vi "Sys config window-Get set control values.vi"(8 "error in (no error)":errorcluster, 11 "Function":T33) -> (0 "error out":errorcluster, 3 "output cluster":T1={"Triggers output setup"=[], "General trigger settings"={"Trigger 1 function"=enum."Encoder trigger", "Triggers loop clock (MHz)"=80.0}, "Calibration settings"={"Pockels cal.Zoom"=0, "Pockels cal.Dwell time (µs)"=0.0}, "Hardware Configuration"={"Dev. PC"=FALSE, "Swap XY on stage"=FALSE, "No of AOD"=0, "MC Supported"=FALSE, "Axial MC"=FALSE, "Computer MAC address"="", "Externalise Triggers"=FALSE, "Trigger HW config"={"Available Device List"=0, "Device Address"=""}, "DAQmx Chan"={"Pockels AO"="", "Hard shutter AO"="", "PMT AOs"="", "Galvo AOs"="", "Power meter AI"=""}, "XYZ Stage Control Config"=enum."None", "XY stage available"=FALSE, "XY Comms Config Cluster"={"Name"="", "Device Address"="", "Port "=0, "Baudrate"=0, "Comms Type"=enum."GPIB-IEEE488"}, "Y stage available"=FALSE, "Y Comms Config Cluster"={"Name"="", "Device Address"="", "Port "=0, "Baudrate"=0, "Comms Type"=enum."GPIB-IEEE488"}, "Z stage available"=FALSE, "Z Comms Config Cluster "={"Name"="COM7", "Device Address"="", "Port "=0, "Baudrate"=0, "Comms Type"=enum."GPIB-IEEE488"}, "Encoder available"=FALSE, "Encoder"={"IP address"="224.0.1.103", "Port"=7000, "Wheel radius (cm)"=16.0, "Encoder Trigger"=""}, "VidRec available"=FALSE, "Cam VidRec"={"DO flag-Video record"="", "DO flag-Trial start"=""}, "Laser Power Control HW config"={"Laser Power Control"="", "Laser Power Modulation Control"=enum."NI"}, "Laser 1 available"=FALSE, "Laser 1 config cluster"={"COM port"="COM7", "Baud Rate"=0, "Type"=""}, "Prechirper 1 available"=FALSE, "Prechirper 1 config cluster"={"Type"="", "Baud Rate"=0, "COM port"="COM7"}, "Control system.FPGA available?"=FALSE, "Control Sys. HW config"={"Control system.FPGA Type"=enum."Virtex 5", "Control system.Network adapter name"="", "Control system.MAC address"="", "Control system.Ethernet Port"=0, "Control system.Ethernet Port Opened"=FALSE}, "DAQ FPGA HW Config"={"FGPA Ref"=refnum, "Target"="RIO0", "input card type"=enum."AC Card"}, "PMT Control Voltage Limits"={"Lower Limit"=0.0, "Upper Limit"=0.0}}, "System Config"={"Laser wavelength (nm)"=920.0, "DAQ FPGA System"={"Clock Freq (MHz) "=200.0, "Samples Wait after Trigger"=5080, "AOD fill"=4900, "StartupDelay"=0, "Slip Cycle (clock cycles)"=600000, "Add Cycle"=TRUE}, "Control system"={"AOD 1 Amplitude"=0, "AOD 2 Amplitude"=0, "AOD 3 Amplitude"=0, "AOD 4 Amplitude"=0, "AOD 5 Amplitude"=0, "AOD 6 Amplitude"=0, "T0 (ns)"=0.0, "Ta (ns)"=0.0, "Data Time Interval (ns)"=0.0, "Ctrl FPGA Clock (MHz)"=240.0}}, "Calibration config."={"Current Objective"="", "Objective Settings"=[], "PreChirper Values Preset ?"=FALSE, "PreChirper Settings"=[], "PreChirper Constants"={"a 1"=0, "b 1"=0, "c 1"=0, "a 2"=0, "b 2"=0, "c 2"=0, "lmin"=0, "lmax"=0}}, "General Setup"={"Microscope ID"="003", "Microscope Type"="AOLM", "Revision Number"="1.0.0.0", "Advanced Imaging"=FALSE, "Error Logging"=FALSE, "Performance Monitoring"=FALSE, "Max Allowed Trial Length"=60.0, "Initial Scan Resolution"=512.0, "Initial Acceptance Angle"=5.0, "Initial Laser Wavelength"=900.0, "Initial Dwell Time"=900.0}, "AOD Settings - distilled"={"AOD 1 thickness (mm)"=8.0, "AOD 2 thickness (mm)"=8.0, "AOD 3 thickness (mm)"=8.0, "AOD 4 thickness (mm)"=8.0, "AOD 1-2 separation (mm)"=50.0, "AOD 2-3 separation (mm)"=50.0, "AOD 3-4 separation (mm)"=50.0, "AOD 1 Centre (mm)"=7.5, "AOD 2 Centre (mm)"=7.5, "AOD 3 Centre (mm)"=7.5, "AOD 4 Centre (mm)"=7.5, "AOD 1 X Offset"=0.0, "AOD 2 X Offset"=0.0023, "AOD 3 X Offset"=0.0046, "AOD 4 X Offset"=0.0046, "AOD 1 Y Offset"=0.0, "AOD 2 Y Offset"=0.0, "AOD 3 Y Offset"=0.0023, "AOD 4 Y Offset"=0.0046, "Timing Offset AOD 1"=0.0, "Timing Offset AOD 2"=0.0, "Timing Offset AOD 3"=0.0, "Timing Offset AOD 4"=0.0, "AOL centre wavelength (nm)"=1.0, "AOL centre frequency (MHz)"=1.0, "Pair deflection ratio"=1.0, "AOL aperture (mm)"=15.0, "AOD fill time (us)"=1.0, "Diffraction mode"=1.0, "Crystal length (mm)"=0.0, "Acoustic velocity (m/s)"=1.0, "AOD Ord. Refractive index"=2.22}} {"System Config"."Control system"."Ctrl FPGA Clock (MHz)" min=80.0 max=500.0 step=1.0; "System Config"."Control system"."Data Time Interval (ns)" min=0.0 max=2048.0 step=1.0; "System Config"."Control system"."Ta (ns)" min=0.0 max=2048.0 step=1.0; "System Config"."Control system"."T0 (ns)" min=0.0 max=2048.0 step=1.0; "System Config"."Control system"."AOD 6 Amplitude" min=0 max=2048 step=1; "System Config"."Control system"."AOD 5 Amplitude" min=0 max=2048 step=1; "System Config"."Control system"."AOD 4 Amplitude" min=0 max=2048 step=1; "System Config"."Control system"."AOD 3 Amplitude" min=0 max=2048 step=1; "System Config"."Control system"."AOD 2 Amplitude" min=0 max=2048 step=1; "System Config"."Control system"."AOD 1 Amplitude" min=0 max=2048 step=1; "System Config"."Laser wavelength (nm)" min=800.0 max=1080.0 step=1.0; "Hardware Configuration"."Encoder"."Wheel radius (cm)" format="%#_13g"; "General trigger settings"."Triggers loop clock (MHz)" format="%#_13g"; "Triggers output setup"."Pulse width (us)" min=10 max=5000 step=1 format="%.0fµs"})   [LabVIEW 2020]
uses:
  Typedefs/HW config states enum.ctl
  Globals/Sys Config window globals.vi
  Configuration code/Calibration/Globals/gl_Calibration globals.vi
  Configuration code/Typedefs/Pockels Calibration settings cluster.ctl
  Global Variables/General Globals.vi
  Peripherals Control/Triggers/Typedefs/Trigger setup element cluster.ctl
  Peripherals Control/Triggers/Typedefs/Triggers output setup.ctl
  Typedefs/Trigger 1 selector enum.ctl
  Peripherals Control/Triggers/Typedefs/General trigger settings cluster.ctl
  Typedefs/Cam VidRec HW config setup cluster.ctl
  Typedefs/Control Sys HW config cluster.ctl
  <vilib>/userDefined/High Color/nirio_resource_hc.ctl
  Typedefs/FPGA input type AC-DC.ctl
  Typedefs/DAQmx physical channels cluster.ctl
  Typedefs/Encoder config cluster.ctl
  Typedefs/Triggers HW config.ctl
  Typedefs/Laser 1 config cluster.ctl
  Typedefs/PreChirper 1 config cluster.ctl
  Typedefs/Laser Power Control HW config.ctl
  Typedefs/Hardware Configuration settings.ctl
  RIG-SPECIFIC FILES/FPGA Refs/FPGA Ref.ctl
  Typedefs/DAQ FPGA system config.ctl
  Typedefs/CTRL system config.ctl
  Typedefs/System Configuration.ctl
  Configuration code/Typedefs/Initial config.ctl
  Typedefs/PreChirper constants.ctl
  Typedefs/Prechirper Cal Config.ctl
  Typedefs/Objective Config.ctl
  Typedefs/Calibration config.ctl
  Typedefs/fgv_actions.ctl
  Typedefs/General Setup.ctl
  Typedefs/AOD Settings-distilled.ctl
  Typedefs/DAQ FPGA HW config cluster.ctl
  Typedefs/PMT Control Voltage limits.ctl
  Peripherals Control/XYZ Stage/Control/typedefs/XYZControlConfig.ctl
  Typedefs/Comms Type.ctl
  Typedefs/Peripherals comms config cluster.ctl
  Visualisation/Functional Imaging Viewer/Typedefs/Get-Set-Clear Control.ctl
panel:
  # "Thickness (mm)"
  # "X Offset"
  # "Separation (mm)"
  # "Y Offset"
  # "Centre (mm)"
  # "Timing Offset"
  # "(make , model etc)"
  # "(COM Port / IP Address / service address etc.)"
  # "(Port for ethernet / channel for BT)"
  # "(make , model etc)"
  # "(COM Port / IP Address / service address etc.)"
  # "(Port for ethernet / channel for BT)"
  # "(make , model etc)"
  # "(COM Port / IP Address / service address etc.)"
  # "(Port for ethernet / channel for BT)"
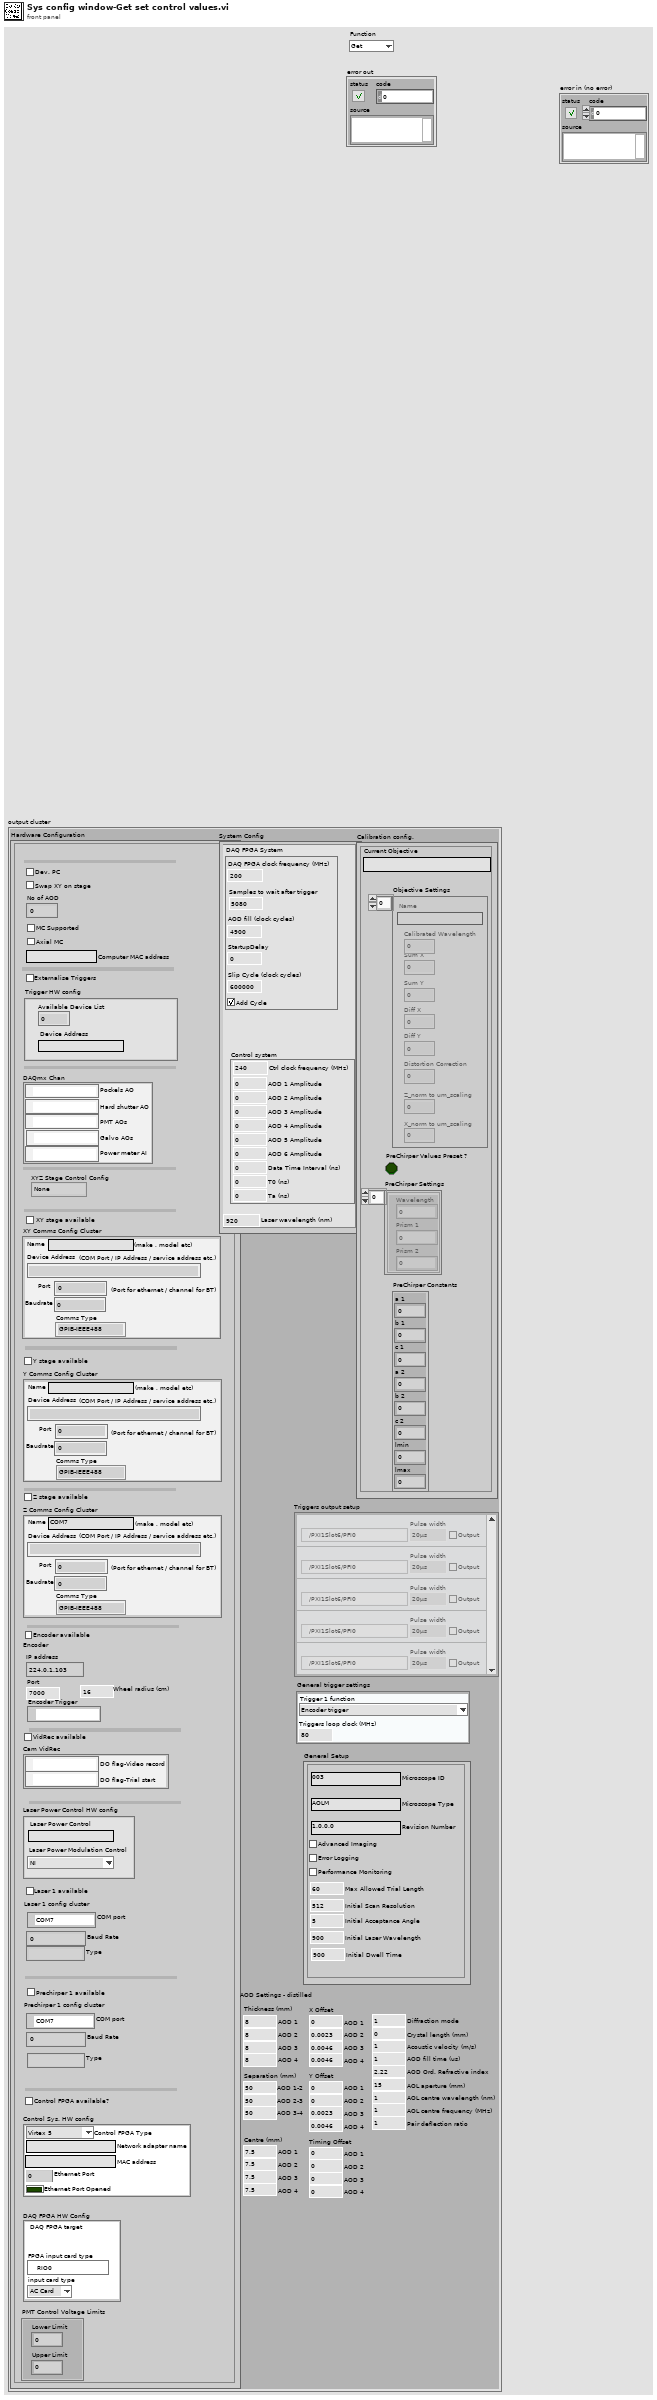
[diagram p1: front panel]
types:
  T1 = typedef "Initial config.ctl" = cluster{"Triggers output setup":T2, "General trigger settings":T4, "Calibration settings":T6, "Hardware Configuration":T7, "System Config":T24, "Calibration config.":T27, "General Setup":T31, "AOD Settings - distilled":T32}
  T2 = typedef "Triggers output setup.ctl" = T3[]
  T3 = typedef "Trigger setup element cluster.ctl" = cluster{"Name":string, "Output?":bool, "Output terminal":tag, "PXI backplane line":tag, "Pulse width (us)":u16}
  T4 = typedef "General trigger settings cluster.ctl" = cluster{"Trigger 1 function":T5, "Triggers loop clock (MHz)":dbl}
  T5 = typedef "Trigger 1 selector enum.ctl" = enum16{"Encoder trigger", "Line trigger", "Control system's ref frame acknowledgement"}
  T6 = typedef "Pockels Calibration settings cluster.ctl" = cluster{"Pockels cal.Zoom":u8, "Pockels cal.Dwell time (µs)":dbl}
  T7 = typedef "Hardware Configuration settings.ctl" = cluster{"Dev. PC":bool, "Swap XY on stage":bool, "No of AOD":u8, "MC Supported":bool, "Axial MC":bool, "Computer MAC address":string, "Externalise Triggers":bool, "Trigger HW config":T8, "DAQmx Chan":T9, "XYZ Stage Control Config":T10, "XY stage available":bool, "XY Comms Config Cluster":T11, "Y stage available":bool, "Y Comms Config Cluster":T11, "Z stage available":bool, "Z Comms Config Cluster ":T11, "Encoder available":bool, "Encoder":T13, "VidRec available":bool, "Cam VidRec":T14, "Laser Power Control HW config":T15, "Laser 1 available":bool, "Laser 1 config cluster":T16, "Prechirper 1 available":bool, "Prechirper 1 config cluster":T17, "Control system.FPGA available?":bool, "Control Sys. HW config":T18, "DAQ FPGA HW Config":T19, "PMT Control Voltage Limits":T23}
  T8 = typedef "Triggers HW config.ctl" = cluster{"Available Device List":i32, "Device Address":string}
  T9 = typedef "DAQmx physical channels cluster.ctl" = cluster{"Pockels AO":tag, "Hard shutter AO":tag, "PMT AOs":tag, "Galvo AOs":tag, "Power meter AI":tag}
  T10 = typedef "XYZControlConfig.ctl" = enum16{"None", "XYZ", "XY-Z", "X-Y-Z", "Z"}
  T11 = typedef "Peripherals comms config cluster.ctl" = cluster{"Name":string, "Device Address":string, "Port ":u16, "Baudrate":i32, "Comms Type":T12}
  T12 = typedef "Comms Type.ctl" = enum16{"GPIB-IEEE488", "Serial-RS232", "Serial-RS485", "Serial-RS422", "Serial-USB", "Ethernet-TCP/IP", "Ethernet-UDP"}
  T13 = typedef "Encoder config cluster.ctl" = cluster{"IP address":string, "Port":u16, "Wheel radius (cm)":dbl, "Encoder Trigger":tag}
  T14 = typedef "Cam VidRec HW config setup cluster.ctl" = cluster{"DO flag-Video record":tag, "DO flag-Trial start":tag}
  T15 = typedef "Laser Power Control HW config.ctl" = cluster{"Laser Power Control":string, "Laser Power Modulation Control":enum16{"NI", "FPGA"}}
  T16 = typedef "Laser 1 config cluster.ctl" = cluster{"COM port":refnum<visa-resource-name>, "Baud Rate":i32, "Type":string}
  T17 = typedef "PreChirper 1 config cluster.ctl" = cluster{"Type":string, "Baud Rate":i32, "COM port":refnum<visa-resource-name>}
  T18 = typedef "Control Sys HW config cluster.ctl" = cluster{"Control system.FPGA Type":enum16{"Virtex 5", "Virtex 7"}, "Control system.Network adapter name":string, "Control system.MAC address":string, "Control system.Ethernet Port":u32, "Control system.Ethernet Port Opened":bool}
  T19 = typedef "DAQ FPGA HW config cluster.ctl" = cluster{"FGPA Ref":T20, "Target":T21, "input card type":T22}
  T20 = typedef "FPGA Ref.ctl" = refnum<k20>
  T21 = typedef "nirio_resource_hc.ctl" = tag
  T22 = typedef "FPGA input type AC-DC.ctl" = enum16{"AC Card", "DC Card"}
  T23 = typedef "PMT Control Voltage limits.ctl" = cluster{"Lower Limit":dbl, "Upper Limit":dbl}
  T24 = typedef "System Configuration.ctl" = cluster{"Laser wavelength (nm)":dbl, "DAQ FPGA System":T25, "Control system":T26}
  T25 = typedef "DAQ FPGA system config.ctl" = cluster{"Clock Freq (MHz) ":dbl, "Samples Wait after Trigger":u16, "AOD fill":u16, "StartupDelay":i32, "Slip Cycle (clock cycles)":u32, "Add Cycle":bool}
  T26 = typedef "CTRL system config.ctl" = cluster{"AOD 1 Amplitude":i16, "AOD 2 Amplitude":i16, "AOD 3 Amplitude":i16, "AOD 4 Amplitude":i16, "AOD 5 Amplitude":i16, "AOD 6 Amplitude":i16, "T0 (ns)":dbl, "Ta (ns)":dbl, "Data Time Interval (ns)":dbl, "Ctrl FPGA Clock (MHz)":dbl}
  T27 = typedef "Calibration config.ctl" = cluster{"Current Objective":string, "Objective Settings":T28[], "PreChirper Values Preset ?":bool, "PreChirper Settings":T29[], "PreChirper Constants":T30}
  T28 = typedef "Objective Config.ctl" = cluster{"Name":string, "Sum X":dbl, "Sum Y":dbl, "Diff X":dbl, "Diff Y":dbl, "Distortion Correction":dbl, "Z_norm to um_scaling":dbl, "X_norm to um_scaling":dbl, "Calibrated Wavelength":dbl}
  T29 = typedef "Prechirper Cal Config.ctl" = cluster{"Wavelength":i32, "Prism 1":i32, "Prism 2":i32}
  T30 = typedef "PreChirper constants.ctl" = cluster{"a 1":i32, "b 1":i32, "c 1":i32, "a 2":i32, "b 2":i32, "c 2":i32, "lmin":i32, "lmax":i32}
  T31 = typedef "General Setup.ctl" = cluster{"Microscope ID":string, "Microscope Type":string, "Revision Number":string, "Advanced Imaging":bool, "Error Logging":bool, "Performance Monitoring":bool, "Max Allowed Trial Length":dbl, "Initial Scan Resolution":dbl, "Initial Acceptance Angle":dbl, "Initial Laser Wavelength":dbl, "Initial Dwell Time":dbl}
  T32 = typedef "AOD Settings-distilled.ctl" = cluster{"AOD 1 thickness (mm)":dbl, "AOD 2 thickness (mm)":dbl, "AOD 3 thickness (mm)":dbl, "AOD 4 thickness (mm)":dbl, "AOD 1-2 separation (mm)":dbl, "AOD 2-3 separation (mm)":dbl, "AOD 3-4 separation (mm)":dbl, "AOD 1 Centre (mm)":dbl, "AOD 2 Centre (mm)":dbl, "AOD 3 Centre (mm)":dbl, "AOD 4 Centre (mm)":dbl, "AOD 1 X Offset":dbl, "AOD 2 X Offset":dbl, "AOD 3 X Offset":dbl, "AOD 4 X Offset":dbl, "AOD 1 Y Offset":dbl, "AOD 2 Y Offset":dbl, "AOD 3 Y Offset":dbl, "AOD 4 Y Offset":dbl, "Timing Offset AOD 1":dbl, "Timing Offset AOD 2":dbl, "Timing Offset AOD 3":dbl, "Timing Offset AOD 4":dbl, "AOL centre wavelength (nm)":dbl, "AOL centre frequency (MHz)":dbl, "Pair deflection ratio":dbl, "AOL aperture (mm)":dbl, "AOD fill time (us)":dbl, "Diffraction mode":dbl, "Crystal length (mm)":dbl, "Acoustic velocity (m/s)":dbl, "AOD Ord. Refractive index":dbl}
  T33 = typedef "Get-Set-Clear Control.ctl" = enum16{"Get", "Set", "Clear"}
  T34 = enum16{"Initialise", "Load from file", "Save to file", "Read", "Write"}
  T35 = typedef "HW config states enum.ctl" = enum16{"Load from file", "Save to file", "Save backup", "Write all", "Read all", "Write XY stage settings", "Write DAQ FPGA settings", "Write Control FPGA settings", "Write Phys Channels", "Write System Config", "Write HW Config", "Save System Config", "Save HW Config", "Clear", "Compare from file"}
  T36 = typedef "HW config window refs cluster.ctl" = cluster{"VI's reference":refnum<vi>, "menu reference":refnum<k9>, "Pane":refnum<vi>, "Config Tab Control":refnum<vi>, "Triggers sub-tab control":refnum<vi>, "Microscope ID":refnum<vi>, "Microscope Type":refnum<vi>, "Revision Number":refnum<vi>, "Advanced Imaging":refnum<vi>, "Max Allowed Trial Length":refnum<vi>, "Initial Scan Resolution":refnum<vi>, "Initial Acceptance Angle":refnum<vi>, "Initial Laser Wavelength [nm] ":refnum<vi>, "Initial Dwell Time [us]":refnum<vi>, "Error Logging":refnum<vi>, "Performance Monitoring":refnum<vi>, "Ctrl FPGA available":refnum<vi>, "Control HW config":refnum<vi>, "Control System Config":refnum<vi>, "General trigger settings":refnum<vi>, "Trigger HW config":refnum<vi>, "Externalise Triggers":refnum<vi>, "[Triggers output setup]":refnum<vi>, "DAQ FPGA HW Config":refnum<vi>, "DAQ FPGA System Config":refnum<vi>, "Pockels AO":refnum<vi>, "Hard shutter AO":refnum<vi>, "PMT AOs":refnum<vi>, "Galvo AO":refnum<vi>, "Power meter AI":refnum<vi>, "PMT Voltage Lower Limit":refnum<vi>, "PMT Voltage Upper Limit":refnum<vi>, "XYZ Stage Control Config":refnum<vi>, "XY stage available":refnum<vi>, "XY Comms Config Cluster":refnum<vi>, "Y stage available":refnum<vi>, "Y Comms Config Cluster":refnum<vi>, "Z stage available":refnum<vi>, "Z Comms Config Cluster":refnum<vi>, "Encoder available":refnum<vi>, "Encoder":refnum<vi>, "Encoder IP address":refnum<vi>, "Encoder port":refnum<vi>, "Wheel radius (cm)":refnum<vi>, "Demo mode":refnum<vi>, "Swap XY on stage":refnum<vi>, "Number of AODs":refnum<vi>, "Axial MC Supported":refnum<vi>, "MC Supported":refnum<vi>, "Computer MAC add.":refnum<vi>, "Cam VidRec available":refnum<vi>, "Cam VidRec":refnum<vi>, "DO flag-Video record":refnum<vi>, "DO flag-Trial start":refnum<vi>, "AOD Settings (distilled)":refnum<vi>, "Pockels cal.Dwell time (µs)":refnum<vi>, "Pockels cal.Zoom":refnum<vi>, "Current Objective":refnum<vi>, "[Obj. Calib. Settings]":refnum<vi>, "Laser Wavelength":refnum<vi>, "Laser Power Control \nHW config":refnum<vi>, "Laser 1 available":refnum<vi>, "Laser 1 config":refnum<vi>, "Prechirper 1 available":refnum<vi>, "Prechirper 1 config":refnum<vi>, "PreChirp Preset Values":refnum<vi>, "[PreChirper Preset \nCalibration Values]":refnum<vi>, "Prechirper Constants":refnum<vi>}
  T37 = typedef "fgv_actions.ctl" = enum16{"Get", "Set"}
  T38 = typedef "AOL Properties Cluster.ctl" = cluster{"AOD 1 thickness (mm)":dbl, "AOD 2 thickness (mm)":dbl, "AOD 3 thickness (mm)":dbl, "AOD 4 thickness (mm)":dbl, "AOD 5 thickness (mm)":dbl, "AOD 6 thickness (mm)":dbl, "AOD 1-2 separation (mm)":dbl, "AOD 2-3 separation (mm)":dbl, "AOD 3-4 separation (mm)":dbl, "AOD 4-5 separation (mm)":dbl, "AOD 5-6 separation (mm)":dbl, "AOD 1 X Offset":dbl, "AOD 2 X Offset":dbl, "AOD 3 X Offset":dbl, "AOD 4 X Offset":dbl, "AOD 1 Y Offset":dbl, "AOD 2 Y Offset":dbl, "AOD 3 Y Offset":dbl, "AOD 4 Y Offset":dbl, "AOD 1 X Direction":dbl, "AOD 2 X Direction":dbl, "AOD 3 X Direction":dbl, "AOD 4 X Direction":dbl, "AOD 1 Y Direction":dbl, "AOD 2 Y Direction":dbl, "AOD 3 Y Direction":dbl, "AOD 4 Y Direction":dbl, "AOD 1 Centre (mm)":dbl, "AOD 2 Centre (mm)":dbl, "AOD 3 Centre (mm)":dbl, "AOD 4 Centre (mm)":dbl, "Timing Offset AOD 1":dbl, "Timing Offset AOD 2":dbl, "Timing Offset AOD 3":dbl, "Timing Offset AOD 4":dbl, "AOD Optical offset 1":dbl, "AOD Optical offset 2":dbl, "AOL aperture (mm)":dbl, "AOL centre wavelength (nm)":dbl, "AOL centre frequency (MHz)":dbl, "Diffraction mode":dbl, "Crystal length (mm)":dbl, "Acoustic velocity (m/s)":dbl, "Pair deflection ratio":dbl, "AOD fill time (us)":dbl, "AOD Ord. Refractive index":dbl, "AOD ExtraOrd. Refractive index":dbl}
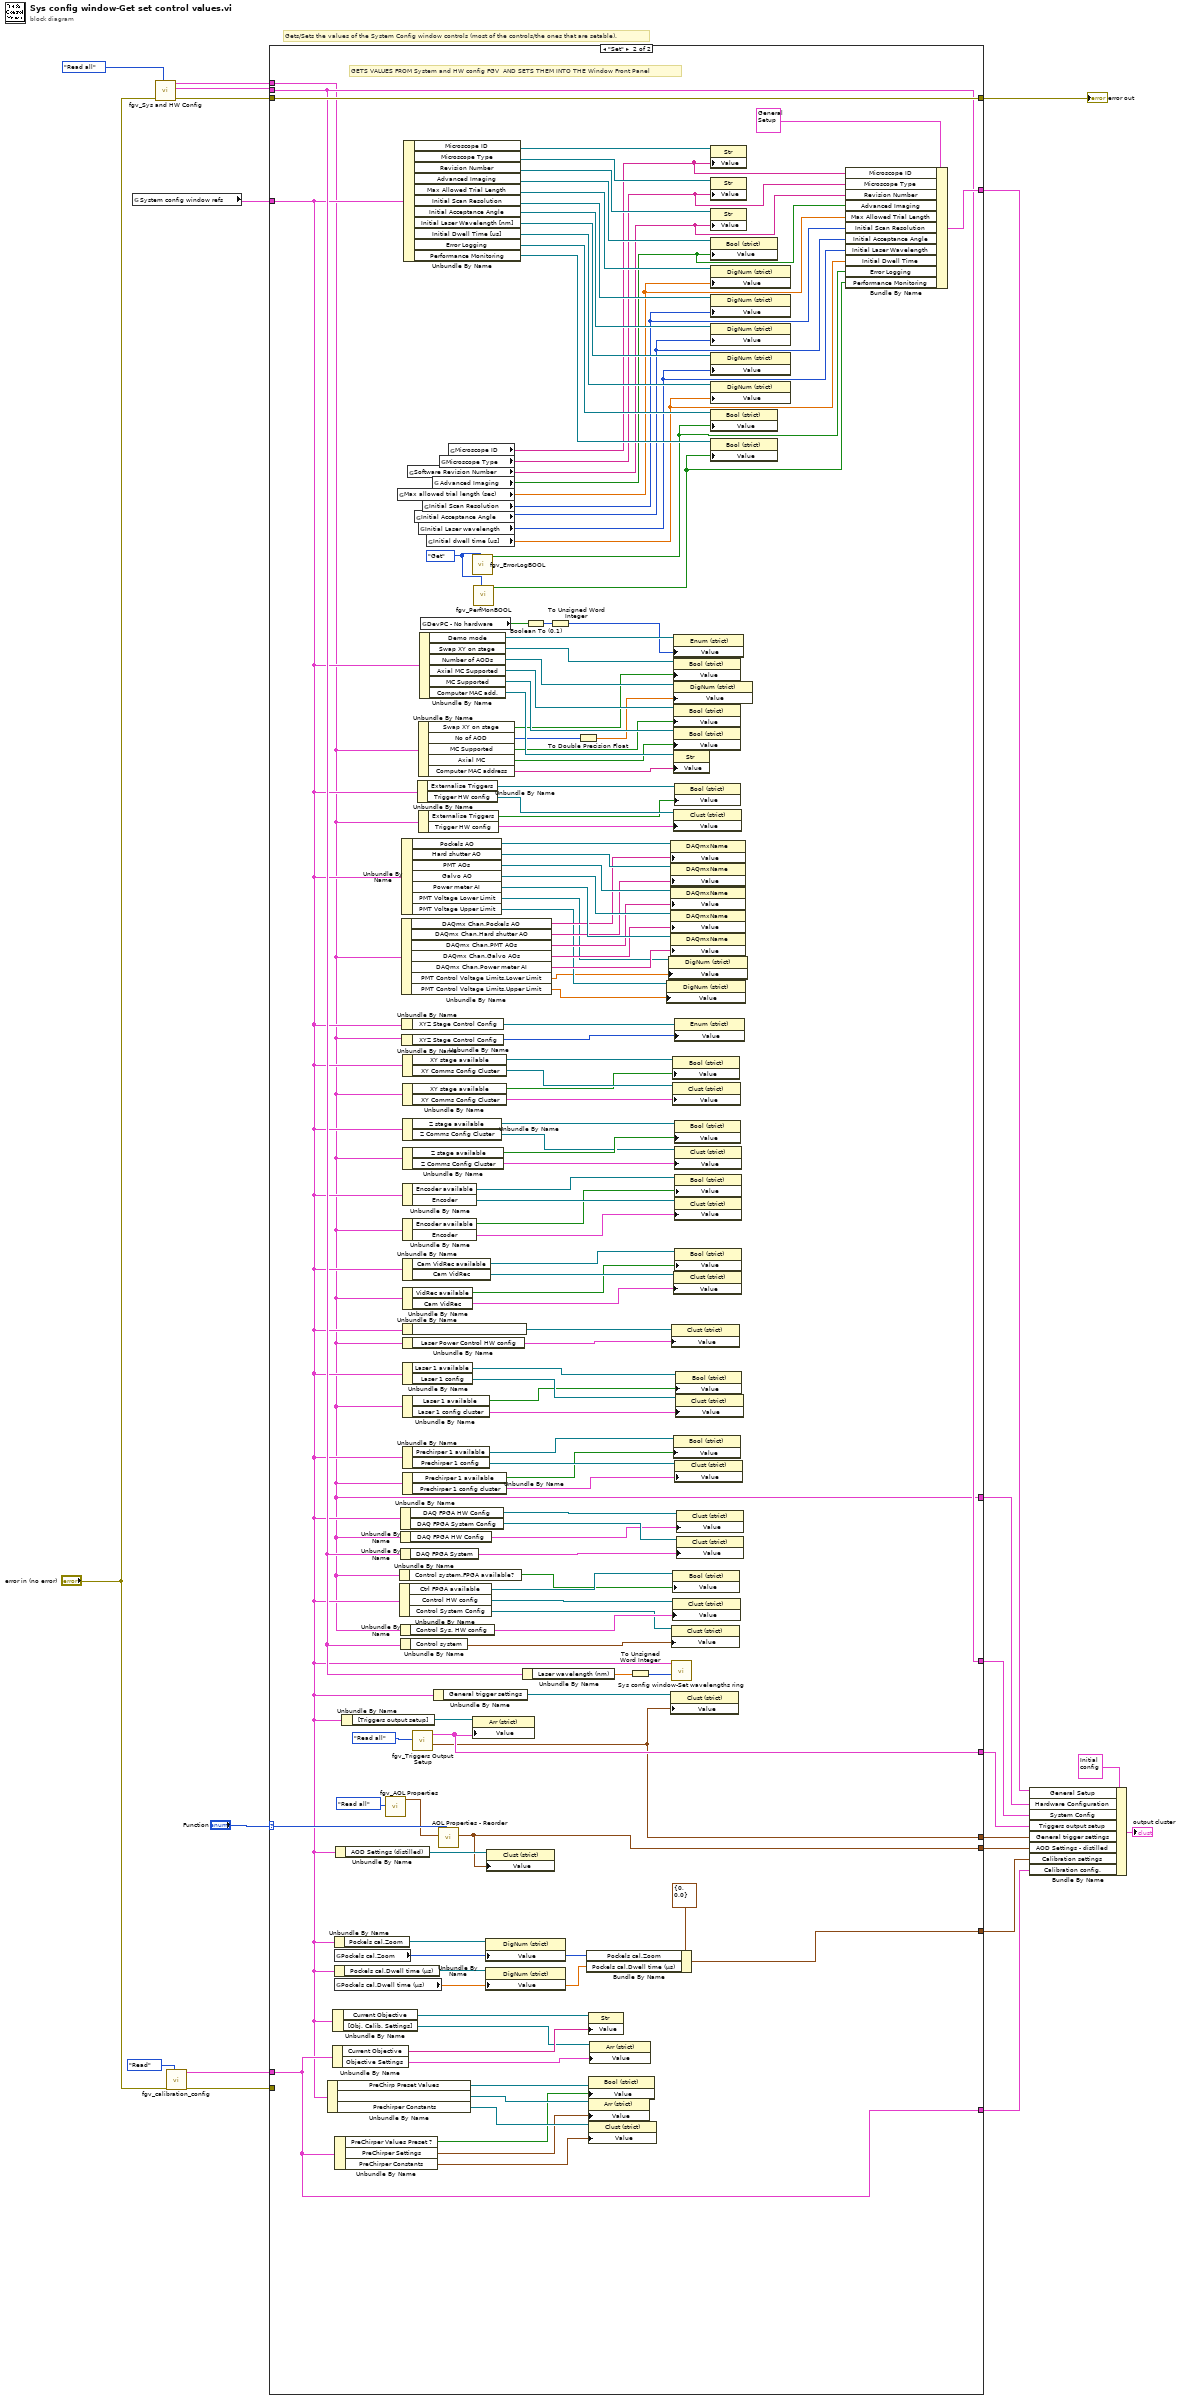
[diagram p0: block diagram]
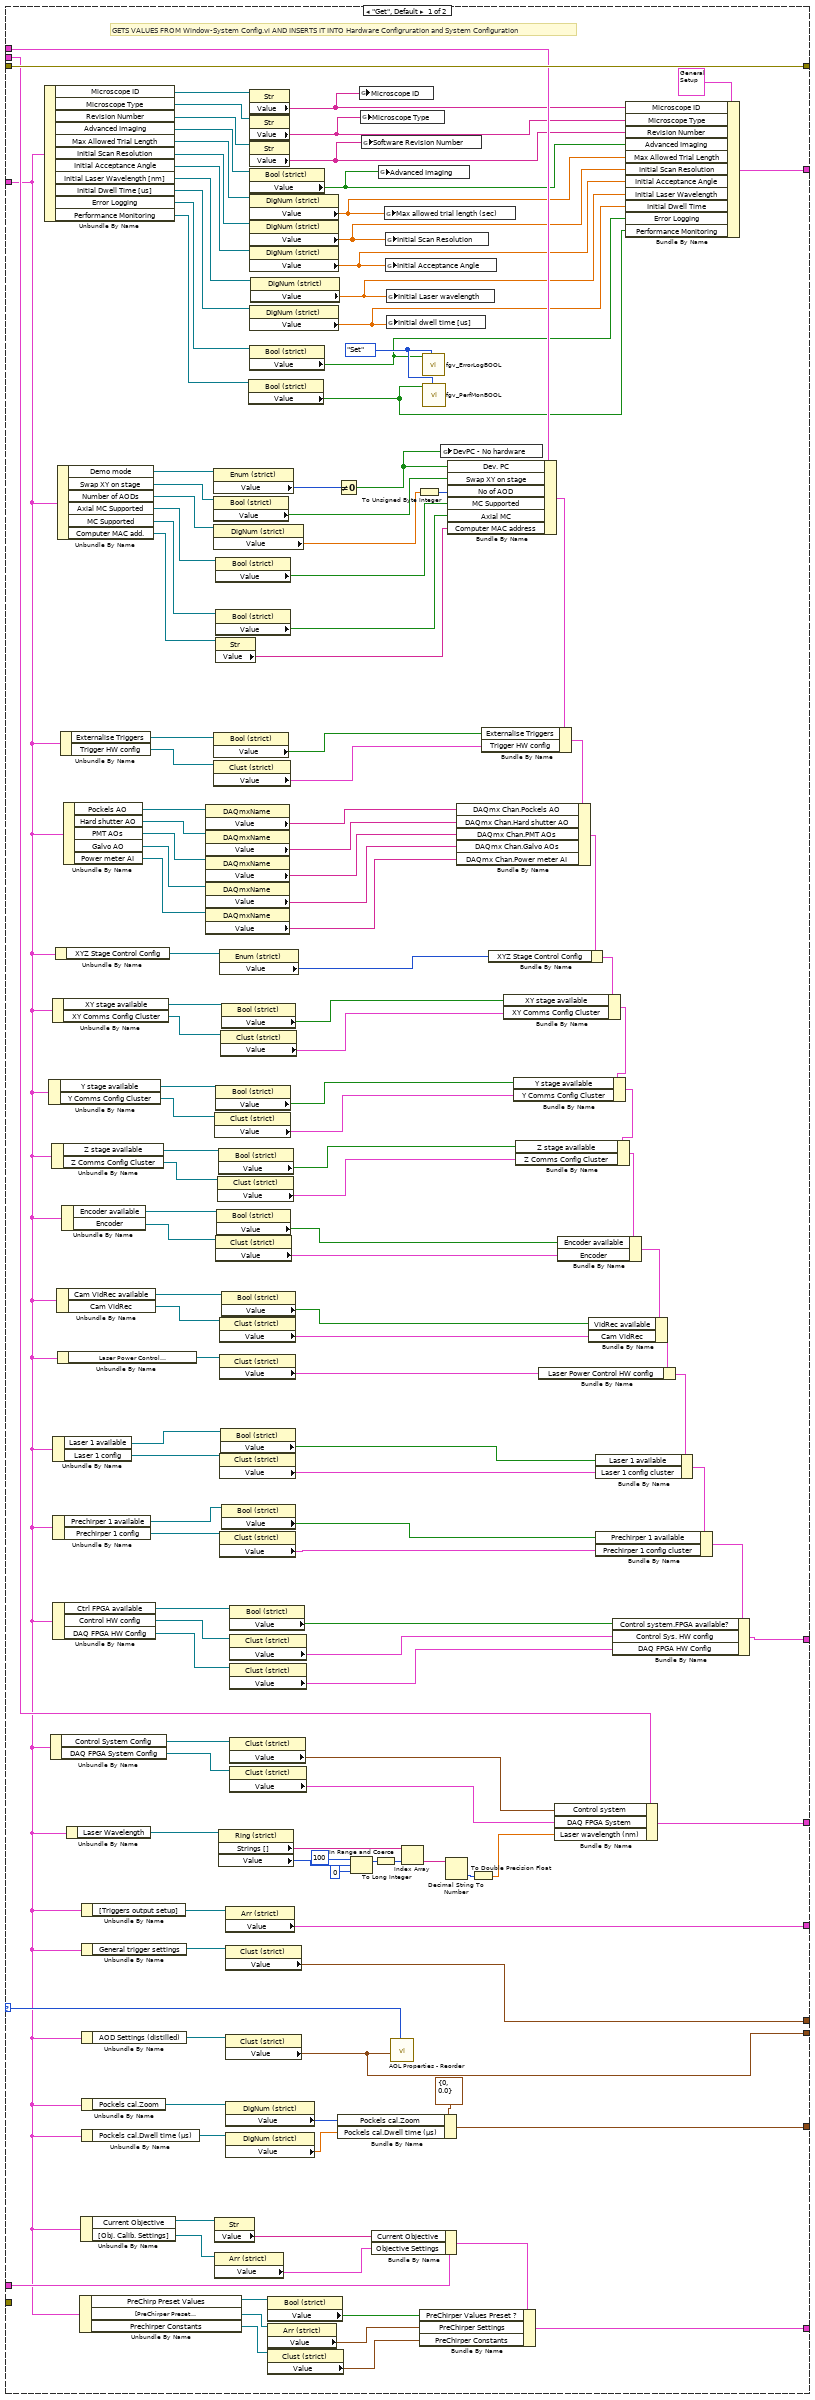
[diagram p2: hidden frame]
diagram:
  # "Gets/Sets the values of the System Config window controls (most of the controls/the ones that are setable)."
  n1 = global read "Sys Config window globals.vi" "System config window refs"() -> (w21:T36)
  n2 = call "fgv_Sys and HW Config.vi"("Function"=HW_config_states_enum."Read all", "error in (no error)"="error in (no error)") -> ("error out"=w16:errorcluster, "System Config OUT"=w13:T24, "Hardware Configuration OUT"=w17:T7)  [unwired: 7 in]
  n3 = call "fgv_calibration_config.vi"("Cal config ops"=T34."Read", "error in (no error)"="error in (no error)") -> ("error out"=w7:errorcluster, "Config cluster OUT"=w8:T27)  [unwired: 7 in, 1 out]
  n4 = case shown="\"Set\"" "Function" {
    selector: "Function" -> [w77 w234]
    tunnel: w21 -> [w24 w176]
    tunnel: [w170 w174] -> w6
    tunnel: [w167 w290] -> w19
    tunnel: [w92 w292] -> w18
    tunnel: w17 -> [w62 w174]
    tunnel: w16 -> [w167 w290]
    tunnel: [w162 w284] -> w15
    tunnel: [w150 w280] -> w14
    tunnel: w13 -> [w94 w182]
    tunnel: w8 -> [w91 w227]
    tunnel: w7 -> [_ _]
    tunnel: [w93 w182] -> w5
    tunnel: [w79 w227] -> w4
    tunnel: [w44 w189] -> w3
    tunnel: [w43 w188] -> w2
    frame "Get", Default {
      w59 = fgv_actions."Set" ("FGV Actions")
      # "GETS VALUES FROM Window-System Config.vi AND INSERTS IT INTO Hardware Configruration and System Configuration"
      n5 = Unbundle By Name(w24) -> ("Microscope ID"=w149:refnum<vi>, "Microscope Type"=w148:refnum<vi>, "Revision Number"=w147:refnum<vi>, "Advanced Imaging"=w146:refnum<vi>, "Max Allowed Trial Length"=w145:refnum<vi>, "Initial Scan Resolution"=w144:refnum<vi>, "Initial Acceptance Angle"=w143:refnum<vi>, "Initial Laser Wavelength [nm]"=w61:refnum<vi>, "Initial Dwell Time [us]"=w60:refnum<vi>, "Error Logging"=w58:refnum<vi>, "Performance Monitoring"=w57:refnum<vi>)
      n6 = Unbundle By Name(w24) -> ("Y stage available"=w27:refnum<vi>, "Y Comms Config Cluster"=w26:refnum<vi>)
      n7 = Unbundle By Name(w24) -> ("Control System Config"=w38:refnum<vi>, "DAQ FPGA System Config"=w36:refnum<vi>)
      n8 = Unbundle By Name(w24) -> ("Z stage available"=w72:refnum<vi>, "Z Comms Config Cluster"=w73:refnum<vi>)
      n9 = Unbundle By Name(w24) -> ("XY stage available"=w113:refnum<vi>, "XY Comms Config Cluster"=w112:refnum<vi>)
      n10 = Unbundle By Name(w24) -> ("Laser 1 available"=w66:refnum<vi>, "Laser 1 config"=w101:refnum<vi>)
      n11 = Unbundle By Name(w24) -> ("Prechirper 1 available"=w64:refnum<vi>, "Prechirper 1 config"=w97:refnum<vi>)
      n12 = Unbundle By Name(w24) -> ("Ctrl FPGA available"=w76:refnum<vi>, "Control HW config"=w42:refnum<vi>, "DAQ FPGA HW Config"=w40:refnum<vi>)
      n13 = Unbundle By Name(w24) -> ("XYZ Stage Control Config"=w32:refnum<vi>)
      n14 = Unbundle By Name(w24) -> ("Cam VidRec available"=w68:refnum<vi>, "Cam VidRec"=w108:refnum<vi>)
      n15 = Unbundle By Name(w24) -> ("Demo mode"=w142:refnum<vi>, "Swap XY on stage"=w141:refnum<vi>, "Number of AODs"=w140:refnum<vi>, "Axial MC Supported"=w135:refnum<vi>, "MC Supported"=w134:refnum<vi>, "Computer MAC add."=w133:refnum<vi>)
      n16 = Unbundle By Name(w24) -> ("Laser Power Control \nHW config"=w104:refnum<vi>)
      n17 = Unbundle By Name(w24) -> ("Externalise Triggers"=w129:refnum<vi>, "Trigger HW config"=w128:refnum<vi>)
      n18 = Unbundle By Name(w24) -> ("Encoder available"=w71:refnum<vi>, "Encoder"=w110:refnum<vi>)
      n19 = Unbundle By Name(w24) -> ("Pockels AO"=w125:refnum<vi>, "Hard shutter AO"=w124:refnum<vi>, "PMT AOs"=w123:refnum<vi>, "Galvo AO"=w122:refnum<vi>, "Power meter AI"=w121:refnum<vi>)
      n20 = Unbundle By Name(w24) -> ("Laser Wavelength"=w161:refnum<vi>)
      n21 = Unbundle By Name(w24) -> ("PreChirp Preset Values"=w85:refnum<vi>, "[PreChirper Preset \nCalibration Values]"=w86:refnum<vi>, "Prechirper Constants"=w84:refnum<vi>)
      n22 = Unbundle By Name(w24) -> ("Current Objective"=w90:refnum<vi>, "[Obj. Calib. Settings]"=w88:refnum<vi>)
      n23 = Unbundle By Name(w24) -> ("[Triggers output setup]"=w169:refnum<vi>)
      n24 = Unbundle By Name(w24) -> ("General trigger settings"=w151:refnum<vi>)
      n25 = Unbundle By Name(w24) -> ("AOD Settings (distilled)"=w168:refnum<vi>)
      n26 = Unbundle By Name(w24) -> ("Pockels cal.Zoom"=w165:refnum<vi>)
      n27 = Unbundle By Name(w24) -> ("Pockels cal.Dwell time (µs)"=w166:refnum<vi>)
      n28 = property class="DAQmxName"(reference=w125) -> ("Value"=w120:string)  [unwired: 1 in, 2 out]
      n29 = property class="DAQmxName"(reference=w124) -> ("Value"=w119:string)  [unwired: 1 in, 2 out]
      n30 = property class="DAQmxName"(reference=w123) -> ("Value"=w118:string)  [unwired: 1 in, 2 out]
      n31 = property class="DAQmxName"(reference=w122) -> ("Value"=w117:string)  [unwired: 1 in, 2 out]
      n32 = property class="DAQmxName"(reference=w121) -> ("Value"=w116:string)  [unwired: 1 in, 2 out]
      n33 = property class="Enum (strict)"(reference=w142) -> ("Value"=w139:enum16{"Full functionality", "Demo mode"})  [unwired: 1 in, 2 out]
      n34 = property class="Bool (strict)"(reference=w141) -> ("Value"=w138:bool)  [unwired: 1 in, 2 out]
      n35 = property class="DigNum (strict)"(reference=w140) -> ("Value"=w136:dbl)  [unwired: 1 in, 2 out]
      n36 = property class="Bool (strict)"(reference=w129) -> ("Value"=w127:bool)  [unwired: 1 in, 2 out]
      n37 = property class="Clust (strict)"(reference=w128) -> ("Value"=w126:T8)  [unwired: 1 in, 2 out]
      n38 = property class="Clust (strict)"(reference=w26) -> ("Value"=w28:T11)  [unwired: 1 in, 2 out]
      n39 = property class="Str"(reference=w90) -> ("Value"=w89:string)  [unwired: 1 in, 2 out]
      n40 = property class="Arr (strict)"(reference=w88) -> ("Value"=w87:T28[])  [unwired: 1 in, 2 out]
      n41 = property class="Bool (strict)"(reference=w135) -> ("Value"=w132:bool)  [unwired: 1 in, 2 out]
      n42 = property class="Bool (strict)"(reference=w134) -> ("Value"=w131:bool)  [unwired: 1 in, 2 out]
      n43 = property class="Str"(reference=w133) -> ("Value"=w130:string)  [unwired: 1 in, 2 out]
      n44 = property class="Bool (strict)"(reference=w27) -> ("Value"=w25:bool)  [unwired: 1 in, 2 out]
      n45 = property class="Clust (strict)"(reference=w110) -> ("Value"=w109:T13)  [unwired: 1 in, 2 out]
      n46 = property class="Bool (strict)"(reference=w71) -> ("Value"=w69:bool)  [unwired: 1 in, 2 out]
      n47 = property class="Clust (strict)"(reference=w73) -> ("Value"=w33:T11)  [unwired: 1 in, 2 out]
      n48 = property class="Bool (strict)"(reference=w72) -> ("Value"=w74:bool)  [unwired: 1 in, 2 out]
      n49 = property on="Property Node" class="Ring (strict)"(reference=w161) -> ("Strings []"=w160:string[], "Value"=w157:u16)  [unwired: 1 in, 2 out]
      n50 = property class="Enum (strict)"(reference=w32) -> ("Value"=w29:T10)  [unwired: 1 in, 2 out]
      n51 = property class="Clust (strict)"(reference=w108) -> ("Value"=w107:T14)  [unwired: 1 in, 2 out]
      n52 = property class="Clust (strict)"(reference=w104) -> ("Value"=w102:T15)  [unwired: 1 in, 2 out]
      n53 = property class="Clust (strict)"(reference=w101) -> ("Value"=w100:T16)  [unwired: 1 in, 2 out]
      n54 = property class="Clust (strict)"(reference=w97) -> ("Value"=w98:T17)  [unwired: 1 in, 2 out]
      n55 = property class="Clust (strict)"(reference=w112) -> ("Value"=w34:T11)  [unwired: 1 in, 2 out]
      n56 = property class="Bool (strict)"(reference=w66) -> ("Value"=w65:bool)  [unwired: 1 in, 2 out]
      n57 = property class="Bool (strict)"(reference=w113) -> ("Value"=w111:bool)  [unwired: 1 in, 2 out]
      n58 = property class="Bool (strict)"(reference=w68) -> ("Value"=w67:bool)  [unwired: 1 in, 2 out]
      n59 = property class="Bool (strict)"(reference=w64) -> ("Value"=w63:bool)  [unwired: 1 in, 2 out]
      n60 = property class="Arr (strict)"(reference=w169) -> ("Value"=w92:T2)  [unwired: 1 in, 2 out]
      n61 = property class="Clust (strict)"(reference=w151) -> ("Value"=w150:T4)  [unwired: 1 in, 2 out]
      n62 = property class="Clust (strict)"(reference=w168) -> ("Value"=w43:T32)  [unwired: 1 in, 2 out]
      n63 = property class="DigNum (strict)"(reference=w165) -> ("Value"=w163:u8)  [unwired: 1 in, 2 out]
      n64 = property class="DigNum (strict)"(reference=w166) -> ("Value"=w164:dbl)  [unwired: 1 in, 2 out]
      n65 = property class="Clust (strict)"(reference=w38) -> ("Value"=w37:T26)  [unwired: 1 in, 2 out]
      n66 = property class="Bool (strict)"(reference=w76) -> ("Value"=w75:bool)  [unwired: 1 in, 2 out]
      n67 = property class="Clust (strict)"(reference=w42) -> ("Value"=w41:T18)  [unwired: 1 in, 2 out]
      n68 = property class="Clust (strict)"(reference=w40) -> ("Value"=w39:T19)  [unwired: 1 in, 2 out]
      n69 = property class="Clust (strict)"(reference=w36) -> ("Value"=w35:T25)  [unwired: 1 in, 2 out]
      n70 = property class="Bool (strict)"(reference=w57) -> ("Value"=w45:bool)  [unwired: 1 in, 2 out]
      n71 = property class="Str"(reference=w149) -> ("Value"=w55:string)  [unwired: 1 in, 2 out]
      n72 = property class="Str"(reference=w148) -> ("Value"=w54:string)  [unwired: 1 in, 2 out]
      n73 = property class="Str"(reference=w147) -> ("Value"=w53:string)  [unwired: 1 in, 2 out]
      n74 = property class="Bool (strict)"(reference=w146) -> ("Value"=w52:bool)  [unwired: 1 in, 2 out]
      n75 = property class="DigNum (strict)"(reference=w145) -> ("Value"=w51:dbl)  [unwired: 1 in, 2 out]
      n76 = property class="DigNum (strict)"(reference=w144) -> ("Value"=w50:dbl)  [unwired: 1 in, 2 out]
      n77 = property class="DigNum (strict)"(reference=w143) -> ("Value"=w49:dbl)  [unwired: 1 in, 2 out]
      n78 = property class="DigNum (strict)"(reference=w60) -> ("Value"=w47:dbl)  [unwired: 1 in, 2 out]
      n79 = property class="Bool (strict)"(reference=w58) -> ("Value"=w46:bool)  [unwired: 1 in, 2 out]
      n80 = property class="DigNum (strict)"(reference=w61) -> ("Value"=w48:dbl)  [unwired: 1 in, 2 out]
      n81 = property class="Bool (strict)"(reference=w85) -> ("Value"=w82:bool)  [unwired: 1 in, 2 out]
      n82 = property class="Arr (strict)"(reference=w86) -> ("Value"=w81:T29[])  [unwired: 1 in, 2 out]
      n83 = property class="Clust (strict)"(reference=w84) -> ("Value"=w80:T30)  [unwired: 1 in, 2 out]
      n84 = Not Equal To 0?(x=w139) -> (x != 0?=w105:bool)
      n85 = Bundle By Name(cluster=T6 {"Pockels cal.Zoom"=0, "Pockels cal.Dwell time (µs)"=0.0} ("Calibration settings"), "Pockels cal.Zoom"=w163, "Pockels cal.Dwell time (µs)"=w164) -> (w162:T6)
      n86 = In Range and Coerce(upper limit=u16 100, x=w157, lower limit=u16 0) -> (coerced(x)=w156:u16)  [unwired: 1 out]
      n87 = global write "General Globals.vi" "Microscope ID"(w55) -> ()
      n88 = global write "General Globals.vi" "Microscope Type"(w54) -> ()
      n89 = global write "General Globals.vi" "Software Revision Number"(w53) -> ()
      n90 = Bundle By Name(cluster=w91, "Current Objective"=w89, "Objective Settings"=w87) -> (w83:T27)
      n91 = To Long Integer(number=w156) -> (32bit integer=w155:i32)
      n92 = global write "General Globals.vi" "Advanced Imaging"(w52) -> ()
      n93 = global write "General Globals.vi" "Max allowed trial length (sec)"(w51) -> ()
      n94 = global write "General Globals.vi" "Initial Scan Resolution"(w50) -> ()
      n95 = global write "General Globals.vi" "Initial Acceptance Angle"(w49) -> ()
      n96 = global write "General Globals.vi" "Initial Laser wavelength"(w48) -> ()
      n97 = global write "General Globals.vi" "Initial dwell time [us]"(w47) -> ()
      n98 = call "AOL Properties - Reorder.vi"("Function"=w77, "Value"=w43) -> ()  [unwired: 8 in, 2 out]
      n99 = Index Array(array=w160, index=w155) -> (element=w153:string)
      n100 = To Unsigned Byte Integer(number=w136) -> (unsigned 8bit integer=w137:u8)
      n101 = Bundle By Name(cluster=w83, "PreChirper Values Preset ?"=w82, "PreChirper Settings"=w81, "PreChirper Constants"=w80) -> (w79:T27)
      n102 = call "fgv_ErrorLogBOOL.vi"("FGV Actions"=w59, "Error Logging ON [IN] ?"=w46) -> ()  [unwired: 8 in, 2 out]
      n103 = call "fgv_PerfMonBOOL.vi"("FGV Actions"=w59, "Perf Mon [IN]"=w45) -> ()  [unwired: 8 in, 2 out]
      n104 = global write "General Globals.vi" "DevPC - No hardware"(w105) -> ()
      n105 = Decimal String To Number(string=w153) -> (number=w152:i32)  [unwired: 2 in, 1 out]
      n106 = Bundle By Name(cluster=w62, "Dev. PC"=w105, "Swap XY on stage"=w138, "No of AOD"=w137, "MC Supported"=w132, "Axial MC"=w131, "Computer MAC address"=w130) -> (w115:T7)
      n107 = To Double Precision Float(number=w152) -> (double precision float=w78:dbl)
      n108 = Bundle By Name(cluster=w115, "Externalise Triggers"=w127, "Trigger HW config"=w126) -> (w114:T7)
      n109 = Bundle By Name(cluster=w114, "DAQmx Chan.Pockels AO"=w120, "DAQmx Chan.Hard shutter AO"=w119, "DAQmx Chan.PMT AOs"=w118, "DAQmx Chan.Galvo AOs"=w117, "DAQmx Chan.Power meter AI"=w116) -> (w31:T7)
      n110 = Bundle By Name(cluster=w31, "XYZ Stage Control Config"=w29) -> (w30:T7)
      n111 = Bundle By Name(cluster=w30, "XY stage available"=w111, "XY Comms Config Cluster"=w34) -> (w23:T7)
      n112 = Bundle By Name(cluster=w23, "Y stage available"=w25, "Y Comms Config Cluster"=w28) -> (w22:T7)
      n113 = Bundle By Name(cluster=w22, "Z stage available"=w74, "Z Comms Config Cluster"=w33) -> (w70:T7)
      n114 = Bundle By Name(cluster=w94, "Control system"=w37, "DAQ FPGA System"=w35, "Laser wavelength (nm)"=w78) -> (w93:T24)
      n115 = Bundle By Name(cluster=w70, "Encoder available"=w69, "Encoder"=w109) -> (w106:T7)
      n116 = Bundle By Name(cluster=w106, "VidRec available"=w67, "Cam VidRec"=w107) -> (w103:T7)
      n117 = Bundle By Name(cluster=w103, "Laser Power Control HW config"=w102) -> (w99:T7)
      n118 = Bundle By Name(cluster=w99, "Laser 1 available"=w65, "Laser 1 config cluster"=w100) -> (w96:T7)
      n119 = Bundle By Name(cluster=w96, "Prechirper 1 available"=w63, "Prechirper 1 config cluster"=w98) -> (w95:T7)
      n120 = Bundle By Name(cluster=w95, "Control system.FPGA available?"=w75, "Control Sys. HW config"=w41, "DAQ FPGA HW Config"=w39) -> (w170:T7)
      n121 = Bundle By Name(cluster=T31 {"Microscope ID"="003", "Microscope Type"="AOLM", "Revision Number"="1.0.0.0", "Advanced Imaging"=FALSE, "Error Logging"=FALSE, "Performance Monitoring"=FALSE, "Max Allowed Trial Length"=60.0, "Initial Scan Resolution"=512.0, "Initial Acceptance Angle"=5.0, "Initial Laser Wavelength"=900.0, "Initial Dwell Time"=900.0} ("Cluster"), "Microscope ID"=w55, "Microscope Type"=w54, "Revision Number"=w53, "Advanced Imaging"=w52, "Max Allowed Trial Length"=w51, "Initial Scan Resolution"=w50, "Initial Acceptance Angle"=w49, "Initial Laser Wavelength"=w48, "Initial Dwell Time"=w47, "Error Logging"=w46, "Performance Monitoring"=w45) -> (w44:T31)
    }
    frame "Set" {
      w202 = fgv_actions."Get" ("FGV Actions")
      # "GETS VALUES FROM System and HW config FGV  AND SETS THEM INTO THE Window Front Panel"
      n122 = Unbundle By Name(w176) -> ("PreChirp Preset Values"=w226:refnum<vi>, "[PreChirper Preset \nCalibration Values]"=w225:refnum<vi>, "Prechirper Constants"=w224:refnum<vi>)
      n123 = Unbundle By Name(w227) -> ("Current Objective"=w228:string, "Objective Settings"=w171:T28[])
      n124 = Unbundle By Name(w176) -> ("Current Objective"=w229:refnum<vi>, "[Obj. Calib. Settings]"=w172:refnum<vi>)
      n125 = Unbundle By Name(w176) -> ("Pockels cal.Zoom"=w288:refnum<vi>)
      n126 = global read "gl_Calibration globals.vi" "Pockels cal.Zoom"() -> (w286:u8)
      n127 = Unbundle By Name(w176) -> ("Pockels cal.Dwell time (µs)"=w289:refnum<vi>)
      n128 = global read "gl_Calibration globals.vi" "Pockels cal.Dwell time (µs)"() -> (w285:dbl)
      n129 = Unbundle By Name(w227) -> ("PreChirper Values Preset ?"=w223:bool, "PreChirper Settings"=w222:T29[], "PreChirper Constants"=w221:T30)
      n130 = Unbundle By Name(w176) -> ("AOD Settings (distilled)"=w293:refnum<vi>)
      n131 = Unbundle By Name(w176) -> ("[Triggers output setup]"=w296:refnum<vi>)
      n132 = call "fgv_AOL Properties.vi"("Function"=HW_config_states_enum."Read all") -> ("AOL Properties out"=w233:T38)  [unwired: 9 in, 1 out]
      n133 = global read "General Globals.vi" "Max allowed trial length (sec)"() -> (w196:dbl)
      n134 = Unbundle By Name(w174) -> ("Control system.FPGA available?"=w207:bool)
      n135 = Unbundle By Name(w176) -> ("Ctrl FPGA available"=w208:refnum<vi>, "Control HW config"=w291:refnum<vi>, "Control System Config"=w186:refnum<vi>)
      n136 = Unbundle By Name(w176) -> ("DAQ FPGA HW Config"=w298:refnum<vi>, "DAQ FPGA System Config"=w184:refnum<vi>)
      n137 = Unbundle By Name(w174) -> ("DAQ FPGA HW Config"=w183:T19)
      n138 = Unbundle By Name(w182) -> ("DAQ FPGA System"=w181:T25)
      n139 = Unbundle By Name(w174) -> ("Control Sys. HW config"=w187:T18)
      n140 = Unbundle By Name(w182) -> ("Control system"=w185:T26)
      n141 = Unbundle By Name(w174) -> ("DAQmx Chan.Pockels AO"=w251:tag, "DAQmx Chan.Hard shutter AO"=w250:tag, "DAQmx Chan.PMT AOs"=w249:tag, "DAQmx Chan.Galvo AOs"=w248:tag, "DAQmx Chan.Power meter AI"=w247:tag, "PMT Control Voltage Limits.Lower Limit"=w178:dbl, "PMT Control Voltage Limits.Upper Limit"=w177:dbl)
      n142 = Unbundle By Name(w176) -> ("Pockels AO"=w256:refnum<vi>, "Hard shutter AO"=w255:refnum<vi>, "PMT AOs"=w254:refnum<vi>, "Galvo AO"=w253:refnum<vi>, "Power meter AI"=w252:refnum<vi>, "PMT Voltage Lower Limit"=w180:refnum<vi>, "PMT Voltage Upper Limit"=w179:refnum<vi>)
      n143 = Unbundle By Name(w176) -> ("XYZ Stage Control Config"=w175:refnum<vi>)
      n144 = Unbundle By Name(w174) -> ("XYZ Stage Control Config"=w173:T10)
      n145 = Unbundle By Name(w176) -> ("XY stage available"=w246:refnum<vi>, "XY Comms Config Cluster"=w245:refnum<vi>)
      n146 = Unbundle By Name(w174) -> ("XY stage available"=w244:bool, "XY Comms Config Cluster"=w243:T11)
      n147 = Unbundle By Name(w176) -> ("Z stage available"=w217:refnum<vi>, "Z Comms Config Cluster"=w218:refnum<vi>)
      n148 = Unbundle By Name(w174) -> ("Z stage available"=w219:bool, "Z Comms Config Cluster"=w220:T11)
      n149 = Unbundle By Name(w176) -> ("Encoder available"=w216:refnum<vi>, "Encoder"=w242:refnum<vi>)
      n150 = Unbundle By Name(w174) -> ("Encoder available"=w215:bool, "Encoder"=w241:T13)
      n151 = Unbundle By Name(w176) -> ("Cam VidRec available"=w214:refnum<vi>, "Cam VidRec"=w240:refnum<vi>)
      n152 = Unbundle By Name(w174) -> ("VidRec available"=w213:bool, "Cam VidRec"=w239:T14)
      n153 = Unbundle By Name(w176) -> ("Laser Power Control \nHW config"=w238:refnum<vi>)
      n154 = Unbundle By Name(w174) -> ("Laser Power Control HW config"=w237:T15)
      n155 = Unbundle By Name(w176) -> ("Laser 1 available"=w212:refnum<vi>, "Laser 1 config"=w299:refnum<vi>)
      n156 = Unbundle By Name(w174) -> ("Laser 1 available"=w211:bool, "Laser 1 config cluster"=w297:T16)
      n157 = Unbundle By Name(w176) -> ("Prechirper 1 available"=w210:refnum<vi>, "Prechirper 1 config"=w235:refnum<vi>)
      n158 = Unbundle By Name(w174) -> ("Prechirper 1 available"=w209:bool, "Prechirper 1 config cluster"=w236:T17)
      n159 = Unbundle By Name(w176) -> ("Microscope ID"=w279:refnum<vi>, "Microscope Type"=w278:refnum<vi>, "Revision Number"=w277:refnum<vi>, "Advanced Imaging"=w276:refnum<vi>, "Max Allowed Trial Length"=w275:refnum<vi>, "Initial Scan Resolution"=w274:refnum<vi>, "Initial Acceptance Angle"=w273:refnum<vi>, "Initial Laser Wavelength [nm]"=w206:refnum<vi>, "Initial Dwell Time [us]"=w205:refnum<vi>, "Error Logging"=w204:refnum<vi>, "Performance Monitoring"=w203:refnum<vi>)
      n160 = global read "General Globals.vi" "Software Revision Number"() -> (w198:string)
      n161 = call "fgv_Triggers Output Setup.vi"("Function"=HW_config_states_enum."Read all") -> ("General trigger settings"=w280:T4, "Triggers output setup"=w292:T2)  [unwired: 8 in, 1 out]
      n162 = global read "General Globals.vi" "Initial Acceptance Angle"() -> (w194:i32)
      n163 = Unbundle By Name(w176) -> ("Externalise Triggers"=w260:refnum<vi>, "Trigger HW config"=w259:refnum<vi>)
      n164 = global read "General Globals.vi" "Initial Laser wavelength"() -> (w193:i32)
      n165 = Unbundle By Name(w174) -> ("Swap XY on stage"=w266:bool, "No of AOD"=w265:u8, "MC Supported"=w263:bool, "Axial MC"=w262:bool, "Computer MAC address"=w261:string)
      n166 = Unbundle By Name(w174) -> ("Externalise Triggers"=w258:bool, "Trigger HW config"=w257:T8)
      n167 = Unbundle By Name(w176) -> ("Demo mode"=w272:refnum<vi>, "Swap XY on stage"=w271:refnum<vi>, "Number of AODs"=w270:refnum<vi>, "Axial MC Supported"=w269:refnum<vi>, "MC Supported"=w268:refnum<vi>, "Computer MAC add."=w267:refnum<vi>)
      n168 = global read "General Globals.vi" "DevPC - No hardware"() -> (w232:bool)
      n169 = global read "General Globals.vi" "Initial Scan Resolution"() -> (w195:i32)
      n170 = global read "General Globals.vi" "Initial dwell time [us]"() -> (w192:dbl)
      n171 = global read "General Globals.vi" "Advanced Imaging"() -> (w197:bool)
      n172 = Unbundle By Name(w176) -> ("General trigger settings"=w281:refnum<vi>)
      n173 = call "AOL Properties - Reorder.vi"("Function"=w234, "AOL Properties out"=w233) -> ("Value"=w188:T32)  [unwired: 8 in, 1 out]
      n174 = global read "General Globals.vi" "Microscope Type"() -> (w199:string)
      n175 = global read "General Globals.vi" "Microscope ID"() -> (w200:string)
      n176 = call "fgv_ErrorLogBOOL.vi"("FGV Actions"=w202) -> ("Error Logging ON [OUT]"=w191:bool)  [unwired: 9 in, 1 out]
      n177 = property class="Arr (strict)"(reference=w296, "Value"=w292) -> ()  [unwired: 1 in, 2 out]
      n178 = call "fgv_PerfMonBOOL.vi"("FGV Actions"=w202) -> ("Perf Mon [OUT]"=w190:bool)  [unwired: 9 in, 1 out]
      n179 = property class="DigNum (strict)"(reference=w288, "Value"=w286) -> ()  [unwired: 1 in, 2 out]
      n180 = property class="DigNum (strict)"(reference=w289, "Value"=w285) -> ()  [unwired: 1 in, 2 out]
      n181 = property class="Clust (strict)"(reference=w293, "Value"=w188) -> ()  [unwired: 1 in, 2 out]
      n182 = Unbundle By Name(w182) -> ("Laser wavelength (nm)"=w283:dbl)
      n183 = Boolean To (0,1)(Boolean=w232) -> (0, 1=w231:i16)
      n184 = To Unsigned Word Integer(number=w231) -> (unsigned 16bit integer=w230:u16)
      n185 = To Double Precision Float(number=w265) -> (double precision float=w264:dbl)
      n186 = Bundle By Name(cluster=T6 {"Pockels cal.Zoom"=0, "Pockels cal.Dwell time (µs)"=0.0} ("Calibration settings"), "Pockels cal.Zoom"=w286, "Pockels cal.Dwell time (µs)"=w285) -> (w284:T6)
      n187 = property class="Str"(reference=w229, "Value"=w228) -> ()  [unwired: 1 in, 2 out]
      n188 = property class="Bool (strict)"(reference=w226, "Value"=w223) -> ()  [unwired: 1 in, 2 out]
      n189 = property class="Arr (strict)"(reference=w225, "Value"=w222) -> ()  [unwired: 1 in, 2 out]
      n190 = property class="Clust (strict)"(reference=w224, "Value"=w221) -> ()  [unwired: 1 in, 2 out]
      n191 = property class="Arr (strict)"(reference=w172, "Value"=w171) -> ()  [unwired: 1 in, 2 out]
      n192 = To Unsigned Word Integer(number=w283) -> (unsigned 16bit integer=w282:u16)
      n193 = property class="DigNum (strict)"(reference=w179, "Value"=w177) -> ()  [unwired: 1 in, 2 out]
      n194 = property class="DigNum (strict)"(reference=w180, "Value"=w178) -> ()  [unwired: 1 in, 2 out]
      n195 = property class="DAQmxName"(reference=w256, "Value"=w251) -> ()  [unwired: 1 in, 2 out]
      n196 = property class="DAQmxName"(reference=w255, "Value"=w250) -> ()  [unwired: 1 in, 2 out]
      n197 = property class="DAQmxName"(reference=w254, "Value"=w249) -> ()  [unwired: 1 in, 2 out]
      n198 = property class="DAQmxName"(reference=w253, "Value"=w248) -> ()  [unwired: 1 in, 2 out]
      n199 = property class="DAQmxName"(reference=w252, "Value"=w247) -> ()  [unwired: 1 in, 2 out]
      n200 = property class="Clust (strict)"(reference=w281, "Value"=w280) -> ()  [unwired: 1 in, 2 out]
      n201 = property class="Clust (strict)"(reference=w238, "Value"=w237) -> ()  [unwired: 1 in, 2 out]
      n202 = property class="Clust (strict)"(reference=w186, "Value"=w185) -> ()  [unwired: 1 in, 2 out]
      n203 = call "Sys config window-Set wavelengths ring.vi"("Laser wavelength (nm)"=w282, "System Config window refs"=w176) -> ()  [unwired: 9 in, 1 out]
      n204 = property class="Clust (strict)"(reference=w291, "Value"=w187) -> ()  [unwired: 1 in, 2 out]
      n205 = property class="Bool (strict)"(reference=w246, "Value"=w244) -> ()  [unwired: 1 in, 2 out]
      n206 = property class="Clust (strict)"(reference=w245, "Value"=w243) -> ()  [unwired: 1 in, 2 out]
      n207 = property class="Bool (strict)"(reference=w208, "Value"=w207) -> ()  [unwired: 1 in, 2 out]
      n208 = property class="Enum (strict)"(reference=w272, "Value"=w230) -> ()  [unwired: 1 in, 2 out]
      n209 = property class="Bool (strict)"(reference=w271, "Value"=w266) -> ()  [unwired: 1 in, 2 out]
      n210 = property class="DigNum (strict)"(reference=w270, "Value"=w264) -> ()  [unwired: 1 in, 2 out]
      n211 = property class="Bool (strict)"(reference=w269, "Value"=w263) -> ()  [unwired: 1 in, 2 out]
      n212 = property class="Bool (strict)"(reference=w268, "Value"=w262) -> ()  [unwired: 1 in, 2 out]
      n213 = property class="Str"(reference=w267, "Value"=w261) -> ()  [unwired: 1 in, 2 out]
      n214 = property class="Clust (strict)"(reference=w259, "Value"=w257) -> ()  [unwired: 1 in, 2 out]
      n215 = property class="Clust (strict)"(reference=w240, "Value"=w239) -> ()  [unwired: 1 in, 2 out]
      n216 = property class="Bool (strict)"(reference=w210, "Value"=w209) -> ()  [unwired: 1 in, 2 out]
      n217 = property class="Bool (strict)"(reference=w260, "Value"=w258) -> ()  [unwired: 1 in, 2 out]
      n218 = property class="Enum (strict)"(reference=w175, "Value"=w173) -> ()  [unwired: 1 in, 2 out]
      n219 = property class="Bool (strict)"(reference=w217, "Value"=w219) -> ()  [unwired: 1 in, 2 out]
      n220 = property class="Clust (strict)"(reference=w218, "Value"=w220) -> ()  [unwired: 1 in, 2 out]
      n221 = property class="Clust (strict)"(reference=w242, "Value"=w241) -> ()  [unwired: 1 in, 2 out]
      n222 = property class="Bool (strict)"(reference=w216, "Value"=w215) -> ()  [unwired: 1 in, 2 out]
      n223 = property class="Bool (strict)"(reference=w214, "Value"=w213) -> ()  [unwired: 1 in, 2 out]
      n224 = property class="Clust (strict)"(reference=w235, "Value"=w236) -> ()  [unwired: 1 in, 2 out]
      n225 = property class="Bool (strict)"(reference=w212, "Value"=w211) -> ()  [unwired: 1 in, 2 out]
      n226 = property class="Clust (strict)"(reference=w299, "Value"=w297) -> ()  [unwired: 1 in, 2 out]
      n227 = property class="Clust (strict)"(reference=w298, "Value"=w183) -> ()  [unwired: 1 in, 2 out]
      n228 = property class="Clust (strict)"(reference=w184, "Value"=w181) -> ()  [unwired: 1 in, 2 out]
      n229 = property class="Str"(reference=w279, "Value"=w200) -> ()  [unwired: 1 in, 2 out]
      n230 = property class="Str"(reference=w278, "Value"=w199) -> ()  [unwired: 1 in, 2 out]
      n231 = property class="Str"(reference=w277, "Value"=w198) -> ()  [unwired: 1 in, 2 out]
      n232 = property class="Bool (strict)"(reference=w276, "Value"=w197) -> ()  [unwired: 1 in, 2 out]
      n233 = property class="DigNum (strict)"(reference=w275, "Value"=w196) -> ()  [unwired: 1 in, 2 out]
      n234 = property class="DigNum (strict)"(reference=w274, "Value"=w195) -> ()  [unwired: 1 in, 2 out]
      n235 = property class="DigNum (strict)"(reference=w273, "Value"=w194) -> ()  [unwired: 1 in, 2 out]
      n236 = property class="DigNum (strict)"(reference=w206, "Value"=w193) -> ()  [unwired: 1 in, 2 out]
      n237 = property class="DigNum (strict)"(reference=w205, "Value"=w192) -> ()  [unwired: 1 in, 2 out]
      n238 = property class="Bool (strict)"(reference=w204, "Value"=w191) -> ()  [unwired: 1 in, 2 out]
      n239 = property class="Bool (strict)"(reference=w203, "Value"=w190) -> ()  [unwired: 1 in, 2 out]
      n240 = Bundle By Name(cluster=T31 {"Microscope ID"="003", "Microscope Type"="AOLM", "Revision Number"="1.0.0.0", "Advanced Imaging"=FALSE, "Error Logging"=FALSE, "Performance Monitoring"=FALSE, "Max Allowed Trial Length"=60.0, "Initial Scan Resolution"=512.0, "Initial Acceptance Angle"=5.0, "Initial Laser Wavelength"=900.0, "Initial Dwell Time"=900.0} ("Cluster"), "Microscope ID"=w200, "Microscope Type"=w199, "Revision Number"=w198, "Advanced Imaging"=w197, "Max Allowed Trial Length"=w196, "Initial Scan Resolution"=w195, "Initial Acceptance Angle"=w194, "Initial Laser Wavelength"=w193, "Initial Dwell Time"=w192, "Error Logging"=w191, "Performance Monitoring"=w190) -> (w189:T31)
    }
  }
  "error out" <- w19
  n241 = Bundle By Name(cluster=T1 {"Triggers output setup"=[], "General trigger settings"={"Trigger 1 function"=enum."Encoder trigger", "Triggers loop clock (MHz)"=0.0}, "Calibration settings"={"Pockels cal.Zoom"=0, "Pockels cal.Dwell time (µs)"=0.0}, "Hardware Configuration"={"Dev. PC"=FALSE, "Swap XY on stage"=FALSE, "No of AOD"=0, "MC Supported"=FALSE, "Axial MC"=FALSE, "Computer MAC address"="", "Externalise Triggers"=FALSE, "Trigger HW config"={"Available Device List"=0, "Device Address"=""}, "DAQmx Chan"={"Pockels AO"="", "Hard shutter AO"="", "PMT AOs"="", "Galvo AOs"="", "Power meter AI"=""}, "XYZ Stage Control Config"=enum."None", "XY stage available"=FALSE, "XY Comms Config Cluster"={"Name"="", "Device Address"="", "Port "=0, "Baudrate"=0, "Comms Type"=enum."GPIB-IEEE488"}, "Y stage available"=FALSE, "Y Comms Config Cluster"={"Name"="", "Device Address"="", "Port "=0, "Baudrate"=0, "Comms Type"=enum."GPIB-IEEE488"}, "Z stage available"=FALSE, "Z Comms Config Cluster "={"Name"="", "Device Address"="", "Port "=0, "Baudrate"=0, "Comms Type"=enum."GPIB-IEEE488"}, "Encoder available"=FALSE, "Encoder"={"IP address"="", "Port"=0, "Wheel radius (cm)"=0.0, "Encoder Trigger"=""}, "VidRec available"=FALSE, "Cam VidRec"={"DO flag-Video record"="", "DO flag-Trial start"=""}, "Laser Power Control HW config"={"Laser Power Control"="", "Laser Power Modulation Control"=enum."NI"}, "Laser 1 available"=FALSE, "Laser 1 config cluster"={"COM port"="", "Baud Rate"=0, "Type"=""}, "Prechirper 1 available"=FALSE, "Prechirper 1 config cluster"={"Type"="", "Baud Rate"=0, "COM port"=""}, "Control system.FPGA available?"=FALSE, "Control Sys. HW config"={"Control system.FPGA Type"=enum."Virtex 5", "Control system.Network adapter name"="", "Control system.MAC address"="", "Control system.Ethernet Port"=0, "Control system.Ethernet Port Opened"=FALSE}, "DAQ FPGA HW Config"={"FGPA Ref"=refnum, "Target"="", "input card type"=enum."AC Card"}, "PMT Control Voltage Limits"={"Lower Limit"=0.0, "Upper Limit"=0.0}}, "System Config"={"Laser wavelength (nm)"=0.0, "DAQ FPGA System"={"Clock Freq (MHz) "=0.0, "Samples Wait after Trigger"=0, "AOD fill"=0, "StartupDelay"=0, "Slip Cycle (clock cycles)"=0, "Add Cycle"=FALSE}, "Control system"={"AOD 1 Amplitude"=0, "AOD 2 Amplitude"=0, "AOD 3 Amplitude"=0, "AOD 4 Amplitude"=0, "AOD 5 Amplitude"=0, "AOD 6 Amplitude"=0, "T0 (ns)"=0.0, "Ta (ns)"=0.0, "Data Time Interval (ns)"=0.0, "Ctrl FPGA Clock (MHz)"=0.0}}, "Calibration config."={"Current Objective"="", "Objective Settings"=[], "PreChirper Values Preset ?"=FALSE, "PreChirper Settings"=[], "PreChirper Constants"={"a 1"=0, "b 1"=0, "c 1"=0, "a 2"=0, "b 2"=0, "c 2"=0, "lmin"=0, "lmax"=0}}, "General Setup"={"Microscope ID"="003", "Microscope Type"="AOLM", "Revision Number"="1.0.0.0", "Advanced Imaging"=FALSE, "Error Logging"=FALSE, "Performance Monitoring"=FALSE, "Max Allowed Trial Length"=60.0, "Initial Scan Resolution"=512.0, "Initial Acceptance Angle"=5.0, "Initial Laser Wavelength"=900.0, "Initial Dwell Time"=900.0}, "AOD Settings - distilled"={"AOD 1 thickness (mm)"=0.0, "AOD 2 thickness (mm)"=0.0, "AOD 3 thickness (mm)"=0.0, "AOD 4 thickness (mm)"=0.0, "AOD 1-2 separation (mm)"=0.0, "AOD 2-3 separation (mm)"=0.0, "AOD 3-4 separation (mm)"=0.0, "AOD 1 Centre (mm)"=0.0, "AOD 2 Centre (mm)"=0.0, "AOD 3 Centre (mm)"=0.0, "AOD 4 Centre (mm)"=0.0, "AOD 1 X Offset"=0.0, "AOD 2 X Offset"=0.0, "AOD 3 X Offset"=0.0, "AOD 4 X Offset"=0.0, "AOD 1 Y Offset"=0.0, "AOD 2 Y Offset"=0.0, "AOD 3 Y Offset"=0.0, "AOD 4 Y Offset"=0.0, "Timing Offset AOD 1"=0.0, "Timing Offset AOD 2"=0.0, "Timing Offset AOD 3"=0.0, "Timing Offset AOD 4"=0.0, "AOL centre wavelength (nm)"=0.0, "AOL centre frequency (MHz)"=0.0, "Pair deflection ratio"=0.0, "AOL aperture (mm)"=0.0, "AOD fill time (us)"=0.0, "Diffraction mode"=0.0, "Crystal length (mm)"=0.0, "Acoustic velocity (m/s)"=0.0, "AOD Ord. Refractive index"=0.0}} ("Initial configuration"), "General Setup"=w3, "Hardware Configuration"=w6, "System Config"=w5, "Triggers output setup"=w18, "General trigger settings"=w14, "AOD Settings - distilled"=w2, "Calibration settings"=w15, "Calibration config."=w4) -> (→"output cluster":T1)
